vi "e.gate Example - Info.vi"(8 "error in (no error)":errorcluster, 11 "IP Address":string) -> (0 "error out":errorcluster)   [LabVIEW 2016]
uses:
  e.gate Time.ctl
  e.gate Protocol Type.ctl
  e.gate HighSpeedPort Diagnostics Full.vi
panel:
  out "Errorneous Channels":string
  out "Error States":string
  out "Run States":string
  out "General States":string
  in  "New Time":T1
  in  "Accept":bool
  out "Actual Time":T1
  in  "Exit":bool
  # "EXAMPLE - HighSpeedPort online communication"
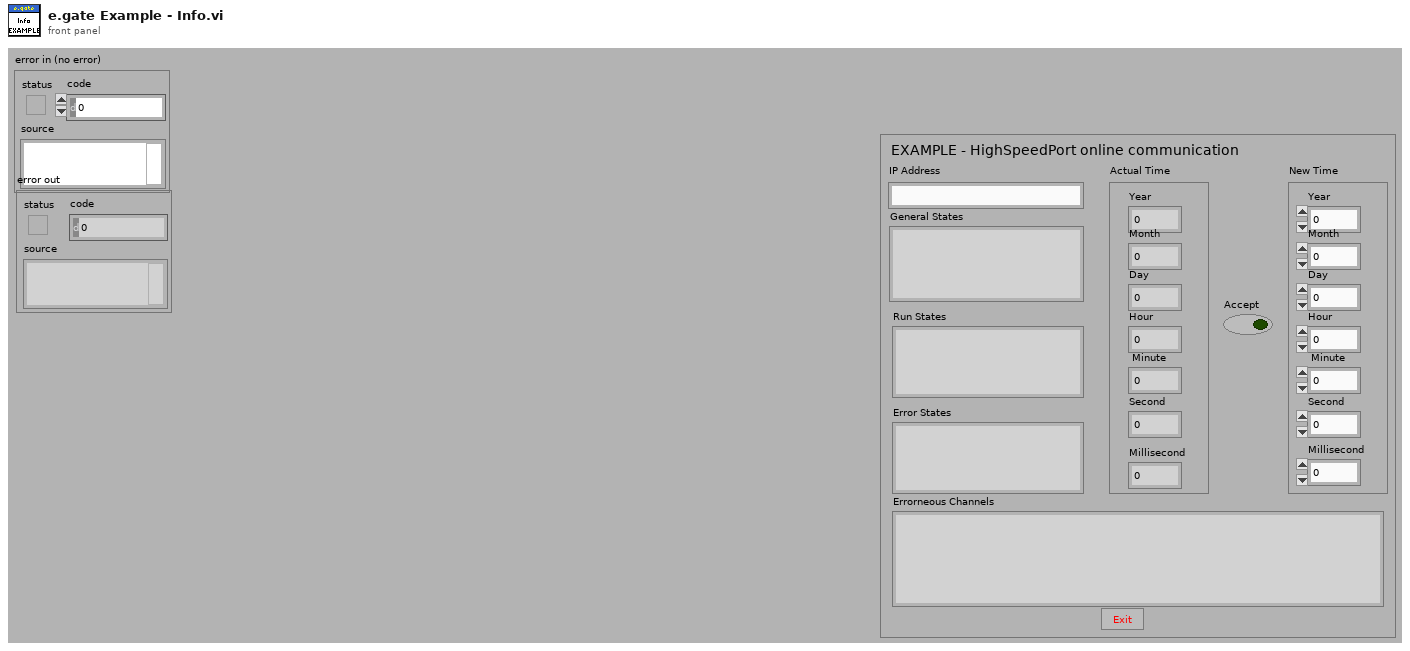
[diagram p1: front panel]
types:
  T1 = typedef "e.gate Time.ctl" = cluster{"Year":dbl, "Month":dbl, "Day":dbl, "Hour":dbl, " Minute":dbl, "Second":dbl, "Millisecond":dbl}
  T2 = typedef "e.gate Protocol Type.ctl" = enum16{"ASCII", "HighspeedPort Online", "HighspeedPort Buffer", "eGateHighspeedPortDLL "}
  T3 = typedef "e.gate Configuration.ctl" = cluster{"connection ID":refnum<k5>, "IPAddress":string, "BufferIndex":i32, "StateMessage":string, "StateCode":i8, "HeaderSize":i32, "BufferSize":i32, "IsBigEndian":i32, "Version":i32, "ChannelCount":i32, "FrameLength":i32, "StartTime":dbl, "dActTimeToSecondFactor":dbl, "StartTimeToDayFactor":dbl, "BufferFillRate":dbl, "SampleRate":dbl, "ChannelData":T4[], "DecodeTimeFormat":string, "SummaryPath":string, "WithCheckSum":i32, "dActTimeDataType":T5, "MaxWriteCount":i32, "MaxReadCount":i32, "TempOffsetRead":i32, "TempLengthRead":i32, "Protocol":T2, "IsSupported":i32, "InputAccessList":i32[], "OutputAccessList":i32[], "DataSource":enum16{"CircleBuffer", "test.con Logger", "test.con Archive"}, "Modules":T6[], "DLL-Handle":T7}
  T4 = typedef "e.gate Channel Data.ctl" = cluster{"VariableName":string, "DataDirection":string, "DataType":string, "DataTypeIndex":T5, "Precision":i16, "FieldLengtht":i16, "ByteCount":i32, "Format":string, "Unit":string, "InputAccessOffset":i32, "OutputAccessOffset":i16, "InputAccessIndex":i16, "OutputAccessIndex":i16, "VarType":string}
  T5 = typedef "e.gate Data Type.ctl" = enum16{"NO", "BOOL", "SINT8", "USINT8", "SINT16", "USINT16", "SINT32", "USINT32", "FLOAT", "SET8", "SET16", "SET32", "DOUBLE", "SINT64", "USINT64", "SET64"}
  T6 = typedef "e.gate Module  Data.ctl" = cluster{"Type":string, "Location":string, "VariablesCount":i16, "UartIndex":i16, "Address":i16, "SystemOffset":i16}
  T7 = typedef "e.gateHSP_DLLhandle.ctl" = cluster{"clientInstance":i32, "connectionInstance":i32}
  T8 = typedef "e.gate Diagnostic Variable Data.ctl" = cluster{"Global Index":i16[], "Error States":i16[]}
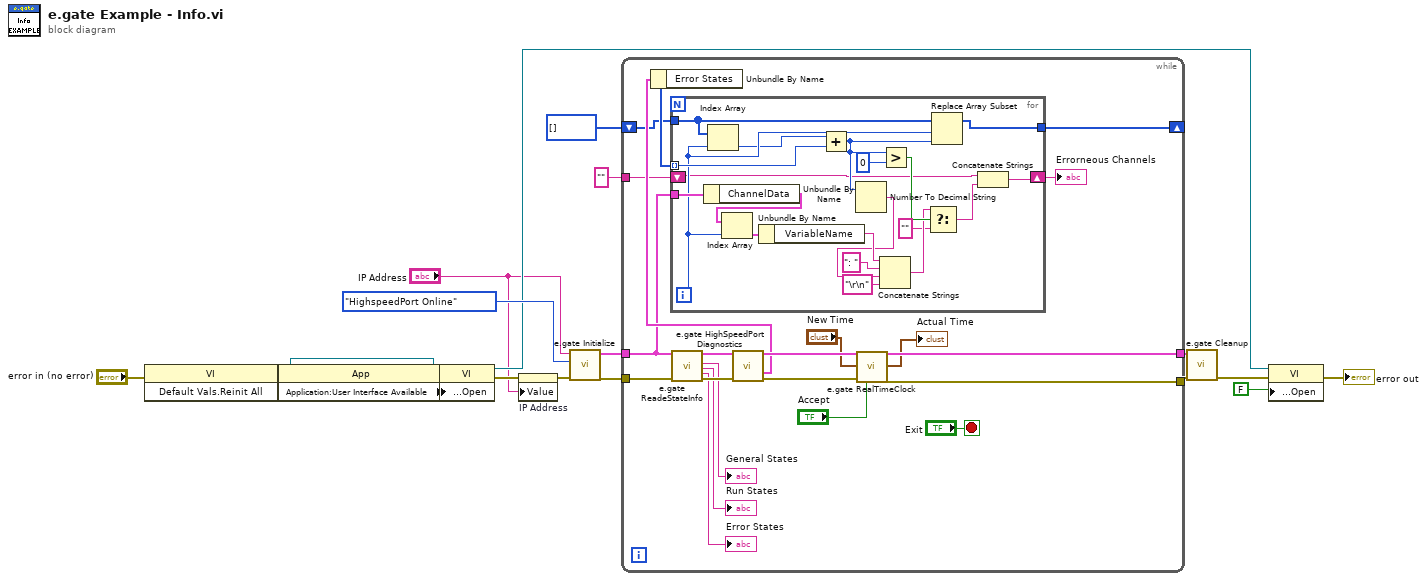
[diagram p0: block diagram]
diagram:
  n1 = invoke class="VI" method="Default Vals.Reinit All"(error in="error in (no error)") -> (reference out=w13:refnum<vi>, error out=w11:errorcluster)  [unwired: 2 in, 1 out]
  n2 = property class="App"(error in=w11) -> (error out=w10:errorcluster, "Application:User Interface Available"=w12:bool)  [unwired: 1 in, 1 out]
  n3 = property class="VI"(reference=w13, error in=w10, "Front Panel.Open"=w12) -> (reference out=w6:refnum<vi>, error out=w3:errorcluster)
  n4 = property on="IP Address" class="Str"(error in=w3, "Value"="IP Address") -> (error out=w2:errorcluster)  [unwired: 1 in, 1 out]
  n5 = call "e.gate Initialize.vi"("error in (no error)"=w2, "Protocol"=e.gate_Protocol_Type."HighspeedPort Online", "IP Address"="IP Address") -> ("error out"=w17:errorcluster, "e.gate Configuration"=w18:T3)  [unwired: 1 in, 6 out]
  n6 = while {
    tunnel: w18 -> [w25]
    tunnel: w17 -> [w40]
    tunnel: [w35] -> w16
    tunnel: [w34] -> w15
    shift-right: [w22] -> _
    shift-left: i16[] [] ("Error States") -> [w23]
    tunnel: "" ("Error States 2") -> [w21]
    stop <- "Exit" stop-if-true
    n7 = call "e.gate ReadeStateInfo.vi"("Configuration  in"=w25, "error in (no error)"=w40) -> ("Configuration out"=w39:T3, "General States"=→"General States":string, "Run States"=→"Run States":string, "Error States"=→"Error States":string, "error out"=w38:errorcluster)  [unwired: 13 out]
    n8 = call-poly "e.gate HighSpeedPort Diagnostics.vi"("e.gate Configuration"=w39, "error in (no error)"=w38) -> ("e.gate Configuration out"=w37:T3, "e.gate Variable Diagnostic Data"=w26:T8, "error out"=w36:errorcluster)  [unwired: 11 out]
    n9 = Unbundle By Name(w26) -> ("Error States"=w24:i16[])
    n10 = for {
      tunnel: w24 -> [w57] mode=indexing
      tunnel: w25 -> [w60]
      tunnel: w23 -> [w55]
      tunnel: [w56] -> w22
      shift-right: [w43] -> w20
      shift-left: w21 -> [w41]
      i -> [w54]
      n11 = Unbundle By Name(w60) -> ("ChannelData"=w59:T4[])
      n12 = Index Array(array=w55, index=w54) -> (element=w53:i16)
      n13 = Index Array(array=w59, index=w54) -> (element=w58:T4)
      n14 = Unbundle By Name(w58) -> ("VariableName"=w49:string)
      n15 = Add(x=w53, y=w57) -> (x+y=w50:i16)
      n16 = Number To Decimal String(number=w50) -> (decimal integer string=w48:string)  [unwired: 1 out]
      n17 = Concatenate Strings(w49, ": " ("String"), w48, "\r\n" ("String")) -> (w45:string)
      n18 = Greater?(x=w50, y=i16 0) -> (0:w51:bool)
      n19 = Select(t=w45, s=w51, f="") -> (s? t:f=w42:string)
      n20 = Replace Array Subset(array=w55, new element=w50, index=w54) -> (w56:i16[])
      n21 = Concatenate Strings(w41, w42) -> (w43:string)
    }
    "Errorneous Channels" <- w20
    n22 = call "e.gate RealTimeClock.vi"("Configuration  in"=w37, "e.gate Time in"="New Time", "error in (no error)"=w36, "Enable writing"="Accept") -> ("Configuration out"=w35:T3, "e.gate Time out"=→"Actual Time":T1, "error out"=w34:errorcluster)  [unwired: 21 out]
  }
  n23 = call "e.gate Cleanup.vi"("error in (no error)"=w15, "e.gate Configuration"=w16) -> ("error out"=w8:errorcluster)  [unwired: 9 out]
  n24 = property class="VI"(reference=w6, error in=w8, "Front Panel.Open"=FALSE ("Frontpanel-Fenster:Öffnen")) -> (error out=→"error out":errorcluster)  [unwired: 1 out]
